vi "File Open Check.vi"(11 "File Path":path) -> (2 "File is open in another application":bool, 3 "File Path Out":path)   [LabVIEW 2019]
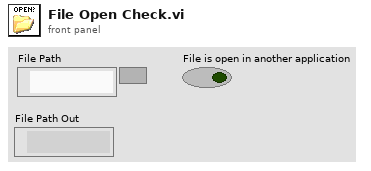
[diagram p1: front panel]
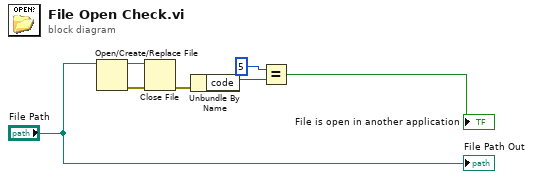
[diagram p0: block diagram]
diagram:
  n1 = Open/Create/Replace File(file path (use dialog)="File Path") -> (refnum out=w3:refnum<file>, error out=w2:errorcluster)  [unwired: 5 in, 1 out]
  n2 = Close File(refnum=w3, error in=w2) -> (error out=w4:errorcluster)  [unwired: 1 out]
  n3 = Unbundle By Name(w4) -> ("code"=w5:i32)
  n4 = Equal?(x=5, y=w5) -> (x = y?=→"File is open in another application":bool)
  "File Path Out" <- "File Path"
